vi "ExQCircBufColor.vi"() -> ()   [LabVIEW 2012]
uses:
  Open-Close/CamHandle.vi
panel:
  in  "Type of Bayer":u32=1 max=4 step=1
  in  "Blue Offset":dbl format="%.2f"
  in  "Green Offset":dbl format="%.2f"
  in  "Red Offset":dbl format="%.2f"
  in  "Blue Gain":dbl=2.17 format="%.2f"
  in  "Red Gain":dbl=1.51 format="%.2f"
  in  "Green Gain":dbl=1.0 format="%.2f"
  in  "Bit shift":u16
  in  "ADC Gain":u32
  out "ADC Speed (Khz)":u32
  in  "Fast ADC":bool=TRUE
  in  "Temperature":dbl format="%.2f"
  in  "Exposure":dbl=0.5 min=0.0 step=0.001 format="%.3f"
  in  "stop":bool
  in  "Store":bool
  out "error out":errorcluster
  in  "error in (no error)":errorcluster
  # "ExCoolSnapCircBufROI:\nThis example allows a single ROI\nto be programmed up. It then runs\nin sync (focus) mode displaying \nthe ROI data as it comes in.\nNote: this example requires the \ncamera support circular buffers.\nThis example also shows how to \nsetup the cascade to run in over-\nlapped mode and how to set the\non-chip multiplication gain and how\nto set the readout port."
  # "NOTICE\n\nTHIS VI USES A GLOBAL CAMERA HANDLE\n\nTHE VI EXOPENGLOBALCAM.VI MUST BE\nRUN AT THE START OF THE WORK SESSION.\nTHE CAMERA WILL REMAIN OPENED.\n\nTHE VI EXCLOSEGLOBALCAM.VI MUST\nBE RUN BEFORE LEAVING LABVIEW."
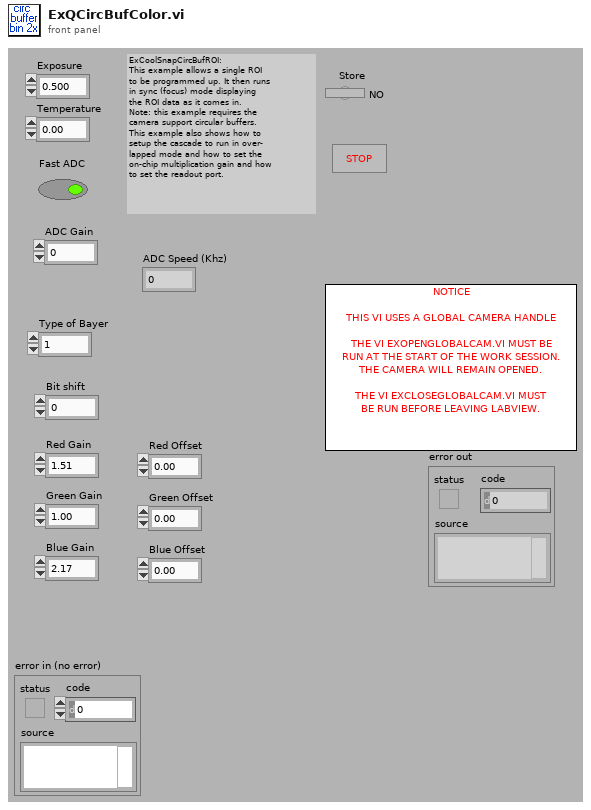
[diagram p1: front panel]
types:
  T1 = cluster{"Type of Bayer":u32, "Red Gain":dbl, "Green Gain":dbl, "Blue Gain":dbl, "Bit shift":u16, "Red Offset":dbl, "Green Offset":dbl, "Blue Offset":dbl}
  T2 = cluster{"acquire focus mode":u32, "Exposure":dbl, "Number of Images":u32, "Software accumulation":u32}
  T3 = cluster{"Camera Handle":u32, "File Handle":u32, "Display Handle":u32, "Image Handle":u32}
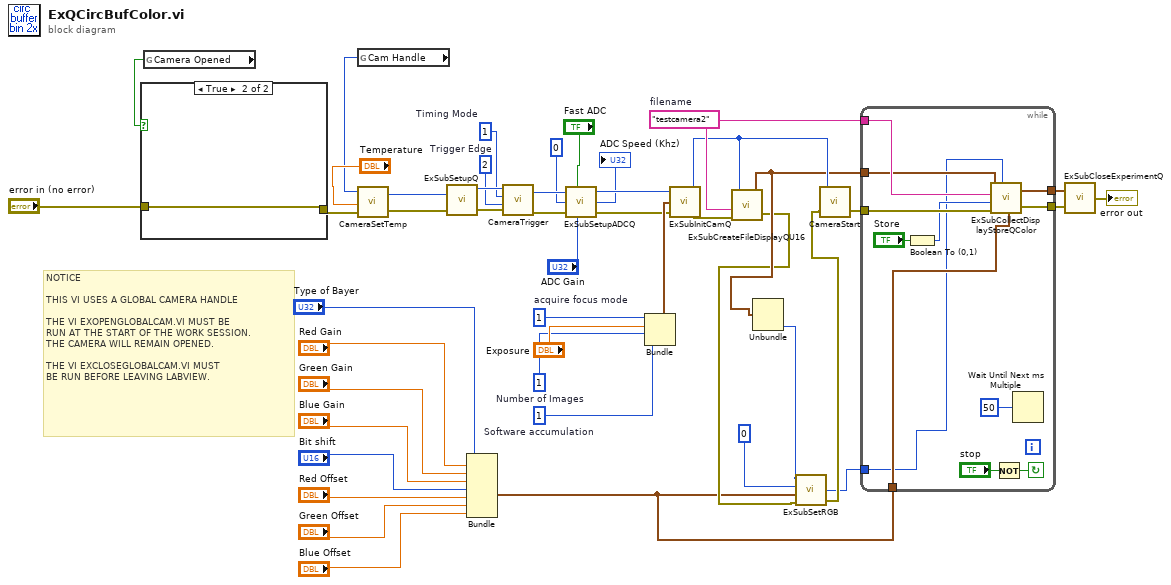
[diagram p0: block diagram]
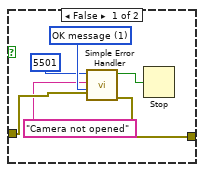
[diagram p2: hidden frame]
diagram:
  w33 = u32 1  # Timing Mode
  w34 = u32 2  # Trigger Edge
  w37 = u32 1  # acquire focus mode
  w36 = u32 1  # Number of Images
  w35 = u32 1  # Software accumulation
  w46 = "testcamera2"  # filename
  # "NOTICE\n\nTHIS VI USES A GLOBAL CAMERA HANDLE\n\nTHE VI EXOPENGLOBALCAM.VI MUST BE\nRUN AT THE START OF THE WORK SESSION.\nTHE CAMERA WILL REMAIN OPENED.\n\nTHE VI EXCLOSEGLOBALCAM.VI MUST\nBE RUN BEFORE LEAVING LABVIEW."
  n1 = global read "CamHandle.vi" "Camera Opened"() -> (w19:bool)
  n2 = case shown="True" w19 {
    tunnel: "error in (no error)" -> [w51 w53]
    tunnel: [w50 w53] -> w20
    frame False {
      w52 = u16 1 items=["no dialog", "OK message", "continue or stop message"] ("type of dialog (OK msg:1)")
      n3 = call <vilib>:"Simple Error Handler.vi"("error code (no error:0)"=5501, "error source (\" \")"="Camera not opened", "type of dialog (OK msg:1)"=w52, "error in (no error)"=w51) -> ("error?"=w48:bool, "error out"=w50:errorcluster)  [unwired: 1 in, 3 out]
      n4 = Stop(stop? (T)=w48) -> ()
    }
    frame True {
    }
  }
  n5 = global read "CamHandle.vi" "Cam Handle"() -> (w18:u32)
  n6 = call <userlib>:"CameraSetTemp.vi"("error in (no error)"=w20, "Temperature"="Temperature", "Camera Handle"=w18) -> ("error out"=w16:errorcluster, "Camera Handle"=w17:u32)
  n7 = call "ExSubSetupQ.vi"("error in (no error)"=w16, "Camera Handle"=w17) -> ("error out"=w30:errorcluster, "Camera Handle"=w39:u32)
  n8 = Bundle("Type of Bayer"="Type of Bayer", "Red Gain"="Red Gain", "Green Gain"="Green Gain", "Blue Gain"="Blue Gain", "Bit shift"="Bit shift", "Red Offset"="Red Offset", "Green Offset"="Green Offset", "Blue Offset"="Blue Offset") -> (w2:T1)  [unwired: 1 in]
  n9 = call <userlib>:"CameraTrigger.vi"("error in"=w30, "Trigger Edge"=w34, "Timing Mode"=w33, "Camera Handle"=w39) -> ("error out"=w28:errorcluster, "Camera Handle"=w29:u32)
  n10 = call "ExSubSetupADCQ.vi"("Camera Handle"=w29, "Fast ADC"="Fast ADC", "ReadOut Port"=0, "error in (no error)"=w28, "ADC Gain"="ADC Gain") -> ("Camera Handle"=w26:u32, "ADC Speed (Khz)"=→"ADC Speed (Khz)":u32, "error out"=w27:errorcluster)
  n11 = Bundle("acquire focus mode"=w37, "Exposure"="Exposure", "Number of Images"=w36, "Software accumulation"=w35) -> (w44:T2)  [unwired: 1 in]
  n12 = call "ExSubInitCamQ.vi"("error in (no error)"=w27, "Camera Information"=w44, "Camera Handle"=w26) -> ("error out"=w43:errorcluster, "Camera Handle"=w32:u32)
  n13 = call "ExSubCreateFileDisplayQU16.vi"("error in (no error)"=w43, "File and Display Name"=w46, "Camera Handle"=w32) -> ("error out"=w4:errorcluster, "Handles Out"=w7:T3)  [unwired: 1 in]
  n14 = Unbundle(w7) -> ("Image Handle"=w5:u32)  [unwired: 3 out]
  n15 = call "ExSubSetRGB.vi"("error in (no error)"=w4, "Adjustments"=w2, "RGB Handle"=0, "Image handle"=w5) -> ("error out"=w3:errorcluster, "RGB handle"=w1:u32)  [unwired: 1 out]
  n16 = call <userlib>:"CameraStart.vi"("error in"=w3, "Camera Handle"=w32) -> ("error out"=w38:errorcluster)  [unwired: 1 out]
  n17 = while {
    tunnel: w7 -> [w56]
    tunnel: w38 -> [w64]
    tunnel: w46 -> [w57]
    tunnel: [w62] -> w41
    tunnel: [w63] -> w42
    tunnel: w2 -> [w55]
    tunnel: w1 -> [w54]
    stop <- w60 continue-if-true
    n18 = Boolean To (0,1)(Boolean="Store") -> (0, 1=w58:i16)
    n19 = call "ExSubCollectDisplayStoreQColor.vi"("Handle Cluster"=w56, "Color Handle"=w54, "Display Title"=w57, "Store flag"=w58, "Adjustments"=w55, "error in (no error)"=w64) -> ("Handle Cluster Out"=w63:T3, "error out"=w62:errorcluster)  [unwired: 1 out]
    n20 = Not(x="stop") -> (.not. x?=w60:bool)
    n21 = Wait Until Next ms Multiple(millisecond multiple=u32 50) -> ()  [unwired: 1 out]
  }
  n22 = call "ExSubCloseExperimentQ.vi"("error in (no error)"=w41, "Handles In"=w42) -> ("error out"=→"error out":errorcluster)
